vi "AMC Local Process Example.vi"() -> ()   [LabVIEW 2017]
panel:
  out "Process":bool
  out "Status":string
  in  "Process":bool
  in  "Exit":bool
  in  "State Variables":cluster{"CurrentFile":path}
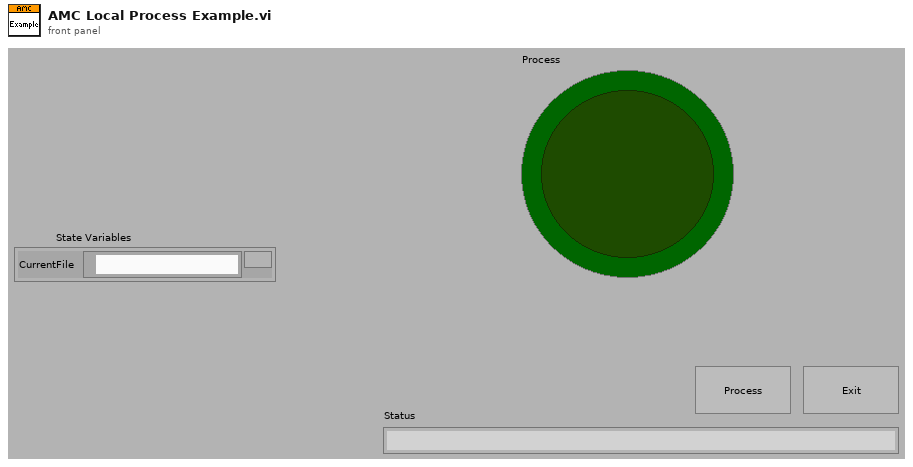
[diagram p1: front panel]
types:
  T1 = typedef "amc_Message Queue.ctl" = refnum<queue>
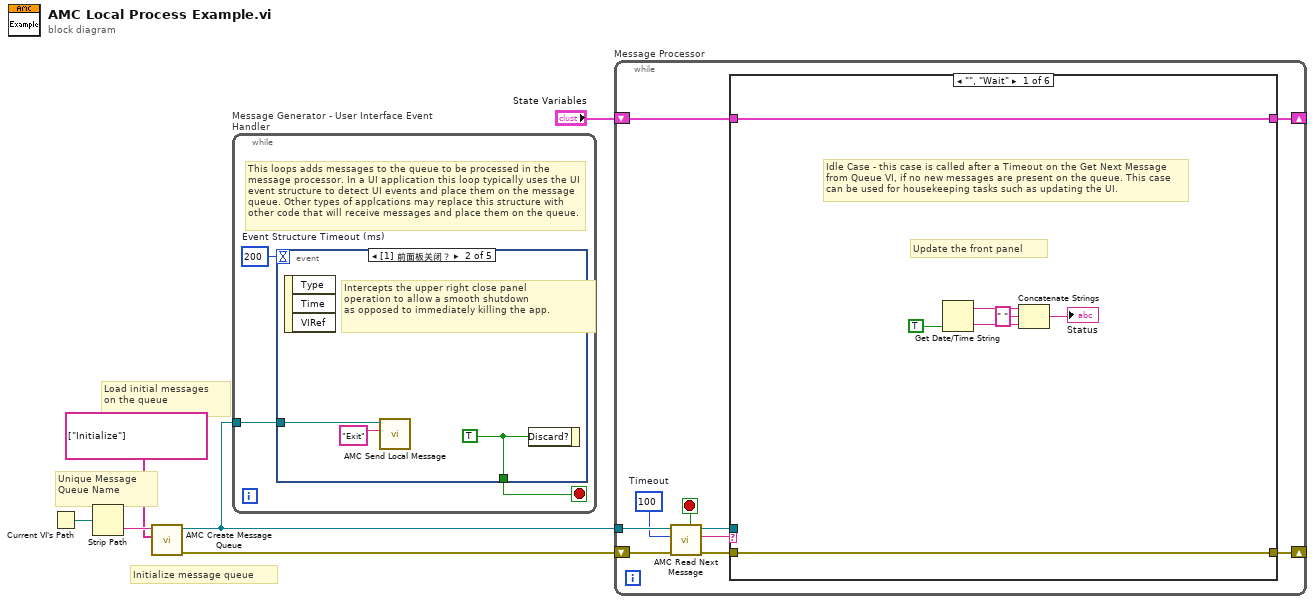
[diagram p0: block diagram]
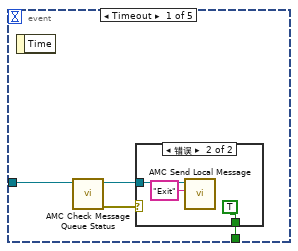
[diagram p2: hidden frame]
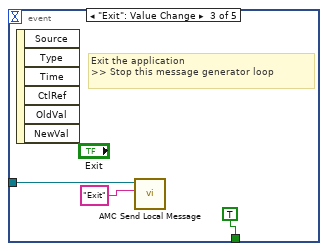
[diagram p4: hidden frame]
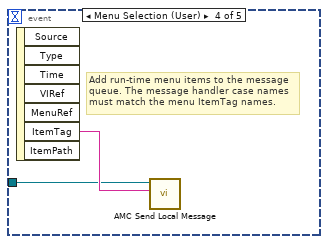
[diagram p5: hidden frame]
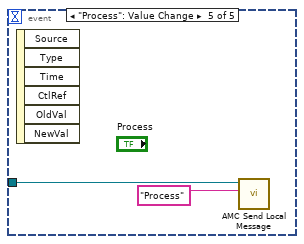
[diagram p6: hidden frame]
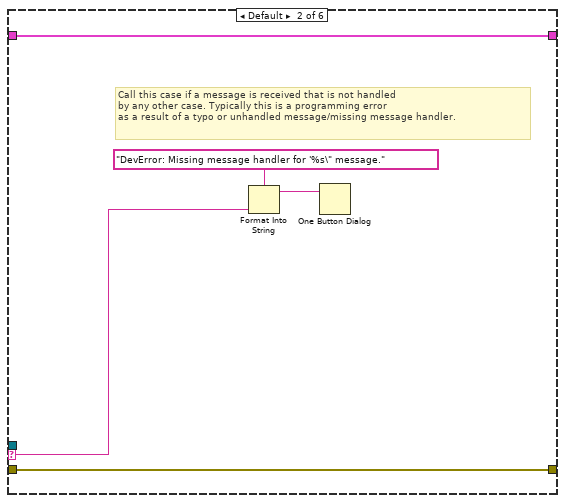
[diagram p7: hidden frame]
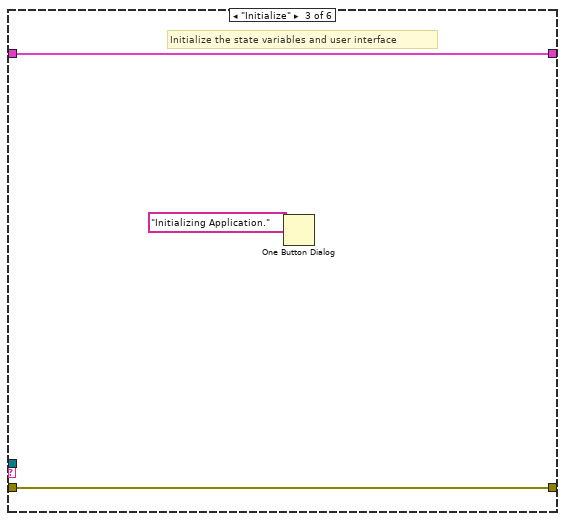
[diagram p8: hidden frame]
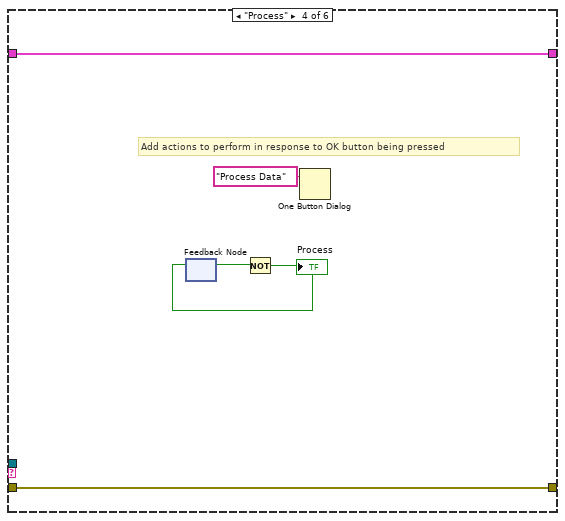
[diagram p9: hidden frame]
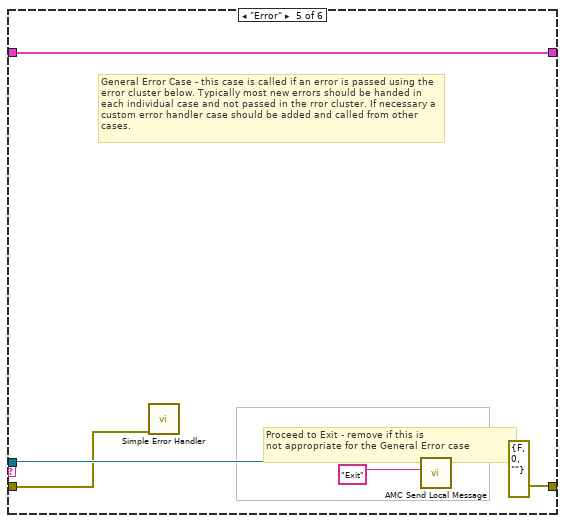
[diagram p10: hidden frame]
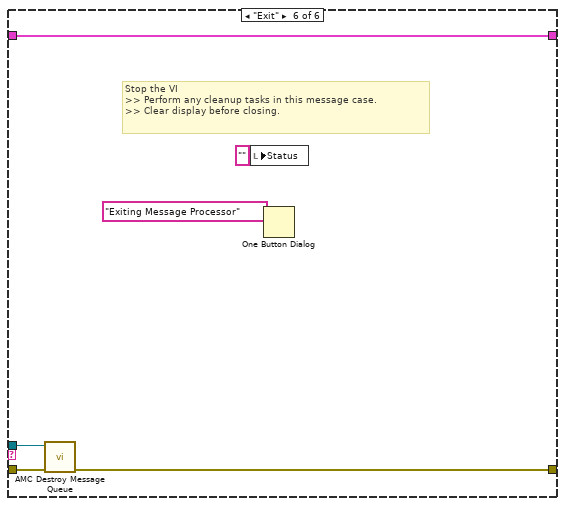
[diagram p11: hidden frame]
diagram:
  # "Initialize message queue"
  # "Unique Message\nQueue Name"
  # "Load initial messages\non the queue"
  n1 = Current VI's Path() -> (path=w5:path)
  n2 = Strip Path(path=w5) -> (name=w6:string)  [unwired: 1 out]
  n3 = call "AMC Create Message Queue.vi"("Initial Message Names"=string[] ["Initialize"], "Message Queue Name"=w6) -> ("error out"=w2:errorcluster, "Message Queue out"=w4:T1)  [unwired: 3 in, 5 out]
  n4 = while "Message Generator - User Interface Event Handler" {
    tunnel: w4 -> [w7]
    stop <- w8 stop-if-true
    w9 = 200  # Event Structure Timeout (ms)
    # "This loops adds messages to the queue to be processed in the message processor. In a UI application this loop typically uses the UI event structure to detect UI events and place them on the message queue. Other types of applcations may replace this structure with other code that will receive messages and place them on the queue."
    n5 = event shown="[1] 前面板关闭？" {
      selector: _ -> [_ _ _ _ _]
      dyn-events: _ -> [_ _ _ _ _]
      timeout: w9 -> [_ _ _ _ _]
      tunnel: [w10 w19 TRUE ("Discard?") _ _] -> w8
      tunnel: w7 -> [w13 w17 w21 w23 w26]
      event Timeout {
        n6 = event-data() -> ()  [unwired: 2 out]
        n7 = call "AMC Check Message Queue Status.vi"("Message queue in"=w13) -> ("error out"=w12:errorcluster, "Message queue out"=w11:T1)  [unwired: 2 in, 6 out]
        n8 = case shown="错误" w12 {
          tunnel: w11 -> [_ w16]
          tunnel: [_ TRUE] -> w10
          frame No Error {
          }
          frame Error {
            n9 = call "AMC Send Local Message.vi"("Message Name"="Exit", "Message Queue in"=w16) -> ()  [unwired: 4 in, 6 out]
          }
        }
      }
      event Panel Close? {
        w19 = TRUE ("Discard?")
        # "Intercepts the upper right close panel\noperation to allow a smooth shutdown\nas opposed to immediately killing the app."
        n10 = event-data() -> ()  [unwired: 4 out]
        n11 = call "AMC Send Local Message.vi"("Message Name"="Exit", "Message Queue in"=w17) -> ()  [unwired: 4 in, 6 out]
        n12 = event-data("Discard?"=w19) -> ()  [unwired: 1 in, 1 out]
      }
      event "Exit": Value Change {
        # "Exit the application\n>> Stop this message generator loop"
        n13 = event-data() -> ()  [unwired: 7 out]
        n14 = call "AMC Send Local Message.vi"("Message Name"="Exit", "Message Queue in"=w21) -> ()  [unwired: 4 in, 6 out]
      }
      event Menu Selection (User) {
        # "Add run-time menu items to the message\nqueue. The message handler case names must match the menu ItemTag names."
        n15 = event-data() -> ("ItemTag"=w24:string)  [unwired: 7 out]
        n16 = call "AMC Send Local Message.vi"("Message Name"=w24, "Message Queue in"=w23) -> ()  [unwired: 4 in, 6 out]
      }
      event "Process": Value Change {
        n17 = event-data() -> ()  [unwired: 7 out]
        n18 = call "AMC Send Local Message.vi"("Message Name"="Process", "Message Queue in"=w26) -> ()  [unwired: 4 in, 6 out]
      }
    }
  }
  n19 = while "Message Processor" {
    shift-left: w2 -> [w31]
    shift-right: [w32] -> _
    tunnel: w4 -> [w30]
    shift-left: "State Variables" -> [w36]
    shift-right: [w35] -> _
    stop <- w29 stop-if-true
    w28 = 100  # Timeout
    n20 = call "AMC Read Next Message.vi"("error in (no error)"=w31, "timeout (1ms)"=w28, "Message Queue in"=w30) -> ("error out"=w33:errorcluster, "Message Name"=w27:string, "Message Queue out"=w34:T1, "Exit Process"=w29:bool)  [unwired: 1 in, 4 out]
    n21 = case shown="\"\", \"Wait\"" w27 {
      selector: w27 -> [_ w46 _ _ _ _]
      tunnel: [w43 w48 w51 w55 w61 w66] -> w35
      tunnel: w36 -> [w43 w48 w51 w55 w61 w66]
      tunnel: w34 -> [_ _ _ _ w59 w63]
      tunnel: w33 -> [w42 w47 w50 w56 w58 w67]
      tunnel: [w42 w47 w50 w56 errorcluster {"status"=FALSE, "code"=0, "source"=""} ("error out") w65] -> w32
      frame "", "Wait" {
        # "Update the front panel"
        # "Idle Case - this case is called after a Timeout on the Get Next Message from Queue VI, if no new messages are present on the queue. This case can be used for housekeeping tasks such as updating the UI."
        n22 = Get Date/Time String(want seconds? (F)=TRUE) -> (date string=w41:string, time string=w40:string)  [unwired: 2 out]
        n23 = Concatenate Strings(w41, " " ("string"), w40) -> (→"Status":string)
      }
      frame Default {
        # "Call this case if a message is received that is not handled \nby any other case. Typically this is a programming error\nas a result of a typo or unhandled message/missing message handler."
        n24 = Format Into String(format string="DevError: Missing message handler for '%s\" message." ("message"), w46) -> (resulting string=w44:string)  [unwired: 2 in, 1 out]
        n25 = One Button Dialog(message=w44) -> ()  [unwired: 2 out]
      }
      frame "Initialize" {
        # "Initialize the state variables and user interface"
        n26 = One Button Dialog(message="Initializing Application.") -> ()  [unwired: 2 out]
      }
      frame "Process" {
        # "Add actions to perform in response to OK button being pressed"
        n27 = feedback #1() -> (w53:bool)  [unwired: 1 out]
        n28 = Not(x=w53) -> (.not. x?=w52:bool)
        "Process" <- w52
        n29 = feedback-in #1(w52) -> ()
        n30 = One Button Dialog(message="Process Data") -> ()  [unwired: 2 out]
      }
      frame "Error" {
        # "Proceed to Exit - remove if this is\nnot appropriate for the General Error case"
        # "General Error Case - this case is called if an error is passed using the error cluster below. Typically most new errors should be handed in each individual case and not passed in the rror cluster. If necessary a custom error handler case should be added and called from other cases."
        n31 = call <vilib>:"Simple Error Handler.vi"("error in (no error)"=w58) -> ()  [unwired: 1 in, 8 out]
        n32 = call "AMC Send Local Message.vi"("Message Name"="Exit", "Message Queue in"=w59) -> ()  [unwired: 4 in, 6 out]
      }
      frame "Exit" {
        # "Stop the VI\n>> Perform any cleanup tasks in this message case.\n>> Clear display before closing."
        n33 = call "AMC Destroy Message Queue.vi"("error in (no error)"=w67, "Message Queue in"=w63) -> ("error out"=w65:errorcluster)  [unwired: 9 out]
        n34 = local write "Status"("" ("Status")) -> ()
        n35 = One Button Dialog(message="Exiting Message Processor" ("button name (\"OK\")")) -> ()  [unwired: 2 out]
      }
    }
  }
